vi "Get RX Received Packets and Bits.vi"(8 "error in (no error)":errorcluster, 11 "niDTS BT Dut in":refnum<class "niDTS BT Dut.lvclass">) -> (0 "error out":errorcluster, 2 "Results":T1, 3 "niDTS BT Dut out":refnum<class "niDTS BT Dut.lvclass">)   [LabVIEW 2015, in "niDTS BT.lvlib" / "niDTS BT Dut.lvclass"]
uses:
  niDTS BT Dut.lvclass
  Tests/Rx Test/Includes/niDTS BT Rx Test INC Results.ctl
  niDTS BT.lvlib
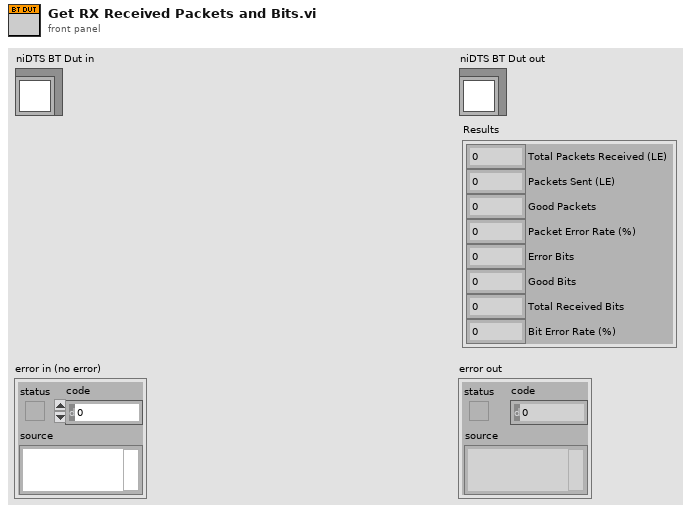
[diagram p1: front panel]
types:
  T1 = typedef "niDTS BT.lvlib/niDTS BT Rx Test INC Results.ctl" = cluster{"Total Packets Received (LE)":i32, "Packets Sent (LE)":dbl, "Good Packets":dbl, "Packet Error Rate (%)":dbl, "Error Bits":u32, "Good Bits":u32, "Total Received Bits":u32, "Bit Error Rate (%)":dbl}
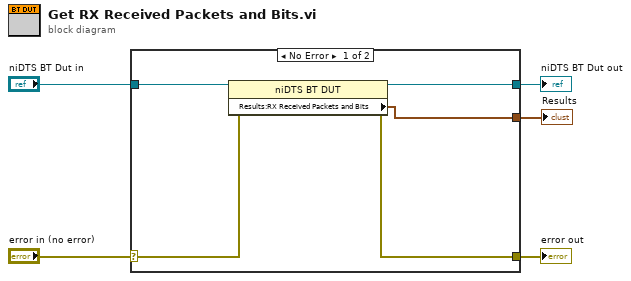
[diagram p0: block diagram]
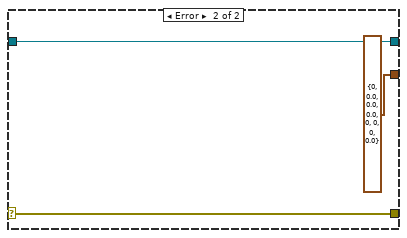
[diagram p2: hidden frame]
diagram:
  n1 = case shown="No Error" "error in (no error)" {
    selector: "error in (no error)" -> [w7 w12]
    tunnel: [w6 w12] -> w4
    tunnel: [w8 w13] -> w2
    tunnel: "niDTS BT Dut in" -> [w9 w13]
    tunnel: [w10 T1 {"Total Packets Received (LE)"=0, "Packets Sent (LE)"=0.0, "Good Packets"=0.0, "Packet Error Rate (%)"=0.0, "Error Bits"=0, "Good Bits"=0, "Total Received Bits"=0, "Bit Error Rate (%)"=0.0} ("Results")] -> w1
    frame No Error {
      n2 = property class="niDTS BT DUT"(reference=w9, error in=w7) -> (reference out=w8:refnum<class "niDTS BT Dut.lvclass">, error out=w6:errorcluster, "Results:RX Received Packets and Bits"=w10:T1)
    }
    frame Error {
    }
  }
  "error out" <- w4
  "niDTS BT Dut out" <- w2
  "Results" <- w1
